vi "Dashboard Main.vi"() -> ()   [LabVIEW 2015]
uses:
  <vilib>/Utility/miscctls.llb/LVRowAndColumnTypeDef.ctl
  <vilib>/event_ctls.llb/eventvkey.ctl
  <vilib>/Rock Robotics/WPI/Dashboard/WPI_DashboardLogging Global.vi
  <vilib>/Rock Robotics/Network Tables/NT Read Boolean.vi
  <vilib>/Rock Robotics/Network Tables/NT Write Boolean.vi
  <vilib>/Utility/config.llb/Write Key (String).vi
  <vilib>/Utility/config.llb/Write Key (I32).vi
  <vilib>/Utility/config.llb/NI_LVConfig.lvlib
panel:
  out "IP Display":string
  in  "TCP":refnum<k5>
  in  "Rec Mode":enum32{"Stop", "Record", "Playback"}(radio)
  in  "Vision":u16(ring)=2 items=["Camera Off", "USB Camera SW", "USB Camera HW", "IP Camera"]
  out "Camera IP":string
  out "Image Message":string="Timeout in Camera Communications"
  in  "Dashboard Tab":T1(tab)
  out "Roll":dbl(slide) scale=0.0..359.0
  out "Pitch":dbl(slide) scale=0.0..359.0
  in  "Select Auto":string(combo)
  out "NT Connection":bool
  in  "Camera Settings":T2={"Frame Rate"=30, "Compression"=30, "Size"=1} {"Frame Rate" scale=1.0..30.0; "Size" items=["640x480", "320x240", "160x120"]}
  out "Gyro":dbl(knob) scale=0.0..360.0
  out "Mode":T3(ring)=enum."Auto Disabled"
  in  "DB Camera Config":bool
  out "fps":dbl format="%#.1g"
  out "Mbps":dbl format="%#.1g"
  out "Mbps LED":bool
  out "isLevel":bool
  out "isGoalCentered":bool
  out "isInSuckState":bool
  out "isOverDefense":bool
  out "Shooter Motors Not Spinning":bool
  out "Script Corrupt?":bool
  out "Com":dbl min=0.0 max=9.0 step=1.0
  out "Auto0":string caption="DB/String 0"
  out "Auto1":string caption="DB/String 1"
  out "Auto2":string caption="DB/String 2"
  out "Auto3":string caption="DB/String 3"
  out "Pos":dbl min=1.0 max=6.0
  out "Script Exists?":bool
  out "Roller Arm State":T4(ring)
  out "Shooter Angle State":T5(ring)
  out "Shooting State":T6(ring)
  out "RollerAngleDesired":dbl
  out "RollerAngleActual":dbl
  out "ShooterAngleDesired":dbl
  out "ShooterAngleActual":dbl
  out "WheelOneDesired":dbl
  out "WheelOneActual":dbl
  out "WheelTwoDesired":dbl
  out "WheelTwoActual":dbl
  in  "doAutoShoot":bool
  in  "ShooterGuideH":i32(slide)=170 min=0 max=320 step=1 scale=0.0..320.0
  in  "ShooterGuideV":i32(slide)=130 caption="ShooterGuide" min=0 max=240 step=1
  in  "Test Slider":dbl(slide) scale=0.0..100.0 scale format="%#_3g"
  in  "On/Off":bool caption="Solenoid"
  in  "Test Name":u16(ring) items=["Select the test to run..."]
  in  "Test Tree":string(tree)
  in  "Motor":cluster{"Value":dbl, "Enable":bool} {"Value" scale=-1.0..1.0 scale format="%#_3g"}
  out "Progress":T7 {"Test Progress" scale=0.0..100.0}
  in  "Rev/Fwd":cluster{"Forward":bool, "Reverse":bool}
  in  "Test Ring":u16(ring) items=["Monochrome", "Color"]
  out "Cmd Status":string
  in  "Execute Command":bool
  in  "Command Params":string[][](table)
  in  "Command Selection":i32(listbox)
  in  "CheckList":i32(listbox)
  out "Tree":string(tree)
  out "Camera Image":T8(plugin-control)
  out "Background":bool
  # "Pitch"
  # "Roll"
  # "D-PAD\n/\\ +Position\n\\/ - Position\n< + Command\n>  - Command"
  # "COMMANDS\n0 - Cross Defense\n1 - Cross Defense, Spit Ball, Return, Spin\n2 - Score Low - Ramp, Moat, Wall, Terrain, Low Bar\n3 - Score High - Ramp, Moat, Wall, Terrain, Low Bar\n4 - Score Low - Cheval de Frise\n5 - Score High - Cheval de Frise\n6 - Score Low - Portcullis\n7 - Score High - Portcullis\n8 - \n9 - \n\nPosition 0 Command 0 - STOP"
  # "POSITION\n0 - Test Scripts\n1 - Defense 1 Low Bar\n2 - Defense 2\n3 - Defense 3\n4 - Defense 4\n5 - Defense 5 Passage\n6 - Spy Box"
  # "Actual"
  # "Desired"
  # "WheelOne"
  # "WheelTwo"
  # "RollerAngle"
  # "ShooterAngle"
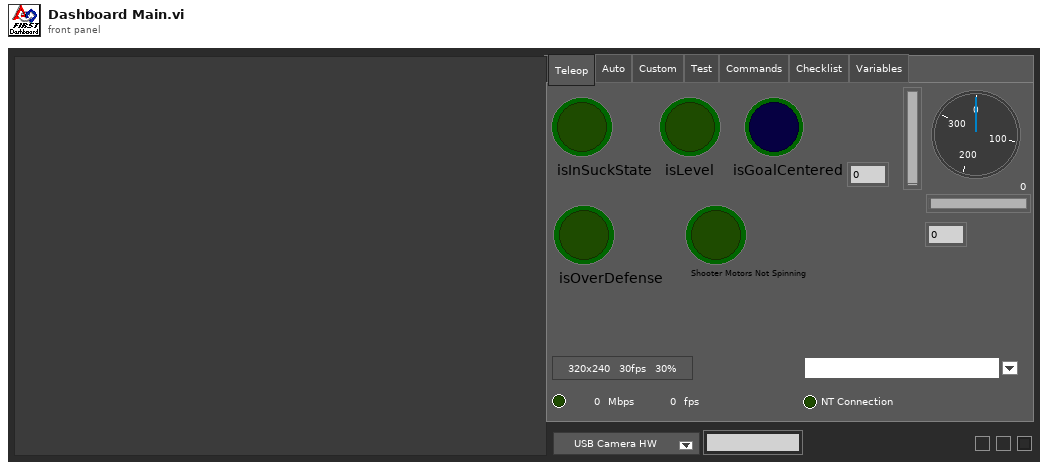
[diagram p1: front panel]
types:
  T1 = enum32{"Teleop", "Auto", "Custom", "Test", "Commands", "Checklist", "Variables"}
  T2 = cluster{"Frame Rate":i32, "Compression":i32, "Size":u16}
  T3 = enum8{"Tele-Op Disabled", "Tele-Op Enabled", "Auto Disabled", "Auto Enabled", "Test Disabled", "Test Enabled", "Disconnected", "No Code", "E-Stop"}
  T4 = enum16{"ResetBack", "EmergencyManualControl", "ResetForward", "Hold", "Reset", "ManualControl"}
  T5 = enum16{"ResetBack", "ResetForward", "Reset", "Hold", "HighGoal", "LowGoal", "BumperShot", "EmergencyManualControl"}
  T6 = enum16{"Empty", "Suck", "Hold", "LowGoal", "HighGoal", "BumperShot", "Shoot", "Dwell"}
  T7 = cluster{"Test Progress":u8, "Test Progress Text":string}
  T8 = typedef "IMAQ Image.ctl" = refnum<image>
  T9 = cluster{"IDs":cluster{"RPC field ID":u16, "Unique ID":u16}, "String":string}
  T10 = enum32{"Drive", "Basic", "Custom", "Test", "Checklist", "Variables"}
  T11 = enum32{"Teleop", "Auto", "Custom", "Test", "Checklist", "Variables"}
  T12 = typedef "Image Type" = u32
  T13 = cluster{"Camera Image":refnum<vi>, "Dashboard Tab":refnum<vi>, "Background":refnum<vi>, "Vision":refnum<vi>, "Rec Mode":refnum<vi>, "Test Slider":refnum<vi>, "On/Off ":refnum<vi>, "Test Ring":refnum<vi>, "Rev/Fwd":refnum<vi>, "Test Name":refnum<vi>, "Motor":refnum<vi>, "Progress":refnum<vi>, "CheckList":refnum<vi>, "Tree":refnum<vi>, "Test Tree":refnum<vi>, "Command Params":refnum<vi>, "Command Selection":refnum<vi>, "Execute Command":refnum<vi>, "Cmd Status":refnum<vi>}
  T14 = cluster{"Error Strings":string, "Disable Counts":cluster{u16, u16}, "Rail Faults":cluster{u16, u16, u16}, "Robot IP":string, "DB Mode":u8, "Event Info":cluster{"Name":string, "Type":u8, "Number":u16, "Replay":u8}, "Camera Addr":string}
  T15 = cluster{"Storage":cluster{"Disk Free":u64, "RAM Block":u32, "RAM free":u32}, "CPU Utilization":cluster{"CPU % ISR":sgl, "CPU % Time Crit":sgl, "CPU % Timed Str":sgl, "CPU % High":sgl, "CPU % Above":sgl, "CPU % Normal":sgl, "CPU % Low":sgl}, "CAN":cluster{"% Bus Utilization":sgl, "Bus Off Cnt":u32, "TX_FIFO Full Cnt":u32, "Receive Error Cnt":u8, "Transmit Error Cnt":u8}, "HID":cluster{"HID Outputs":u32, "Rumble Low":u16, "Rumble High":u16}[]}
  T16 = cluster{"Status bits":cluster{"Test Mode":bool, "Autonomous":bool, "Enabled":bool, "Code Start":bool, "Brownout":bool, "Reserved 2":bool, "Reserved 3":bool, "E-Stop":bool}, "Code Trace":cluster{"Disabled":bool, "TeleOp":bool, "Auto":bool, "Test":bool}, "Controller Type":enum16{"unknown", "cRIO", "roboRio"}, "Code?":enum16{"unknown", "noCode", "code"}, "Battery V":dbl}
  T17 = cluster{"Control Bits":cluster{"TestMode":bool, "Autonomous":bool, "Enabled":bool, "FMS Present":bool, bool, bool, bool, "E-Stop":bool}, "Team Station ":u8, "Countdown":sgl, "Joystick Values":cluster{"Axes":dbl[], "Buttons":bool[], "POVs":i16[]}[]}
  T18 = typedef "NI_LVConfig.lvlib/Config Data RefNum.ctl" = refnum<k1>
  T19 = cluster{"Operation":enum16{"Update", "Clear"}, "Color Box":u32}[]
  T20 = typedef "eventvkey.ctl" = enum16{"ASCII", "Enter", "Return", "Shift", "Ctrl", "Alt", "Cmd", "Opt", "Caps", "NumLock", "Clear", "Break", "Up", "Down", "Left", "Right", "Insert", "Delete", "Home", "End", "PageUp", "PageDown", "Escape", "Help", "Pause", "ScrollLock", "F1", "F2", "F3", "F4", "F5", "F6", "F7", "F8", "F9", "F10", "F11", "F12", "F13", "F14", "F15", "F16", "F17", "F18", "F19", "F20", "F21", "F22", "F23", "F24", "Play", "VolumeUp", "VolumeDown", "Mute", "Two Byte Char"}
  T21 = cluster{"Image Size":bool, "Image Type":bool, "Pixel Value":bool, "ROI Information":bool, "Zoom Factor":bool}
  T22 = enum8{"Enabled", "Disabled", "Disabled and Grayed Out"}
  T23 = cluster{"Operation":enum16{"Update", "Clear"}, "Color Box":u32}
  T24 = typedef "LVRowAndColumnTypeDef.ctl" = cluster{"Row":i32, "Column":i32}
  T25 = cluster{"Shift":bool, "Ctrl":bool, "Alt":bool, "Cmd":bool, "Opt":bool}
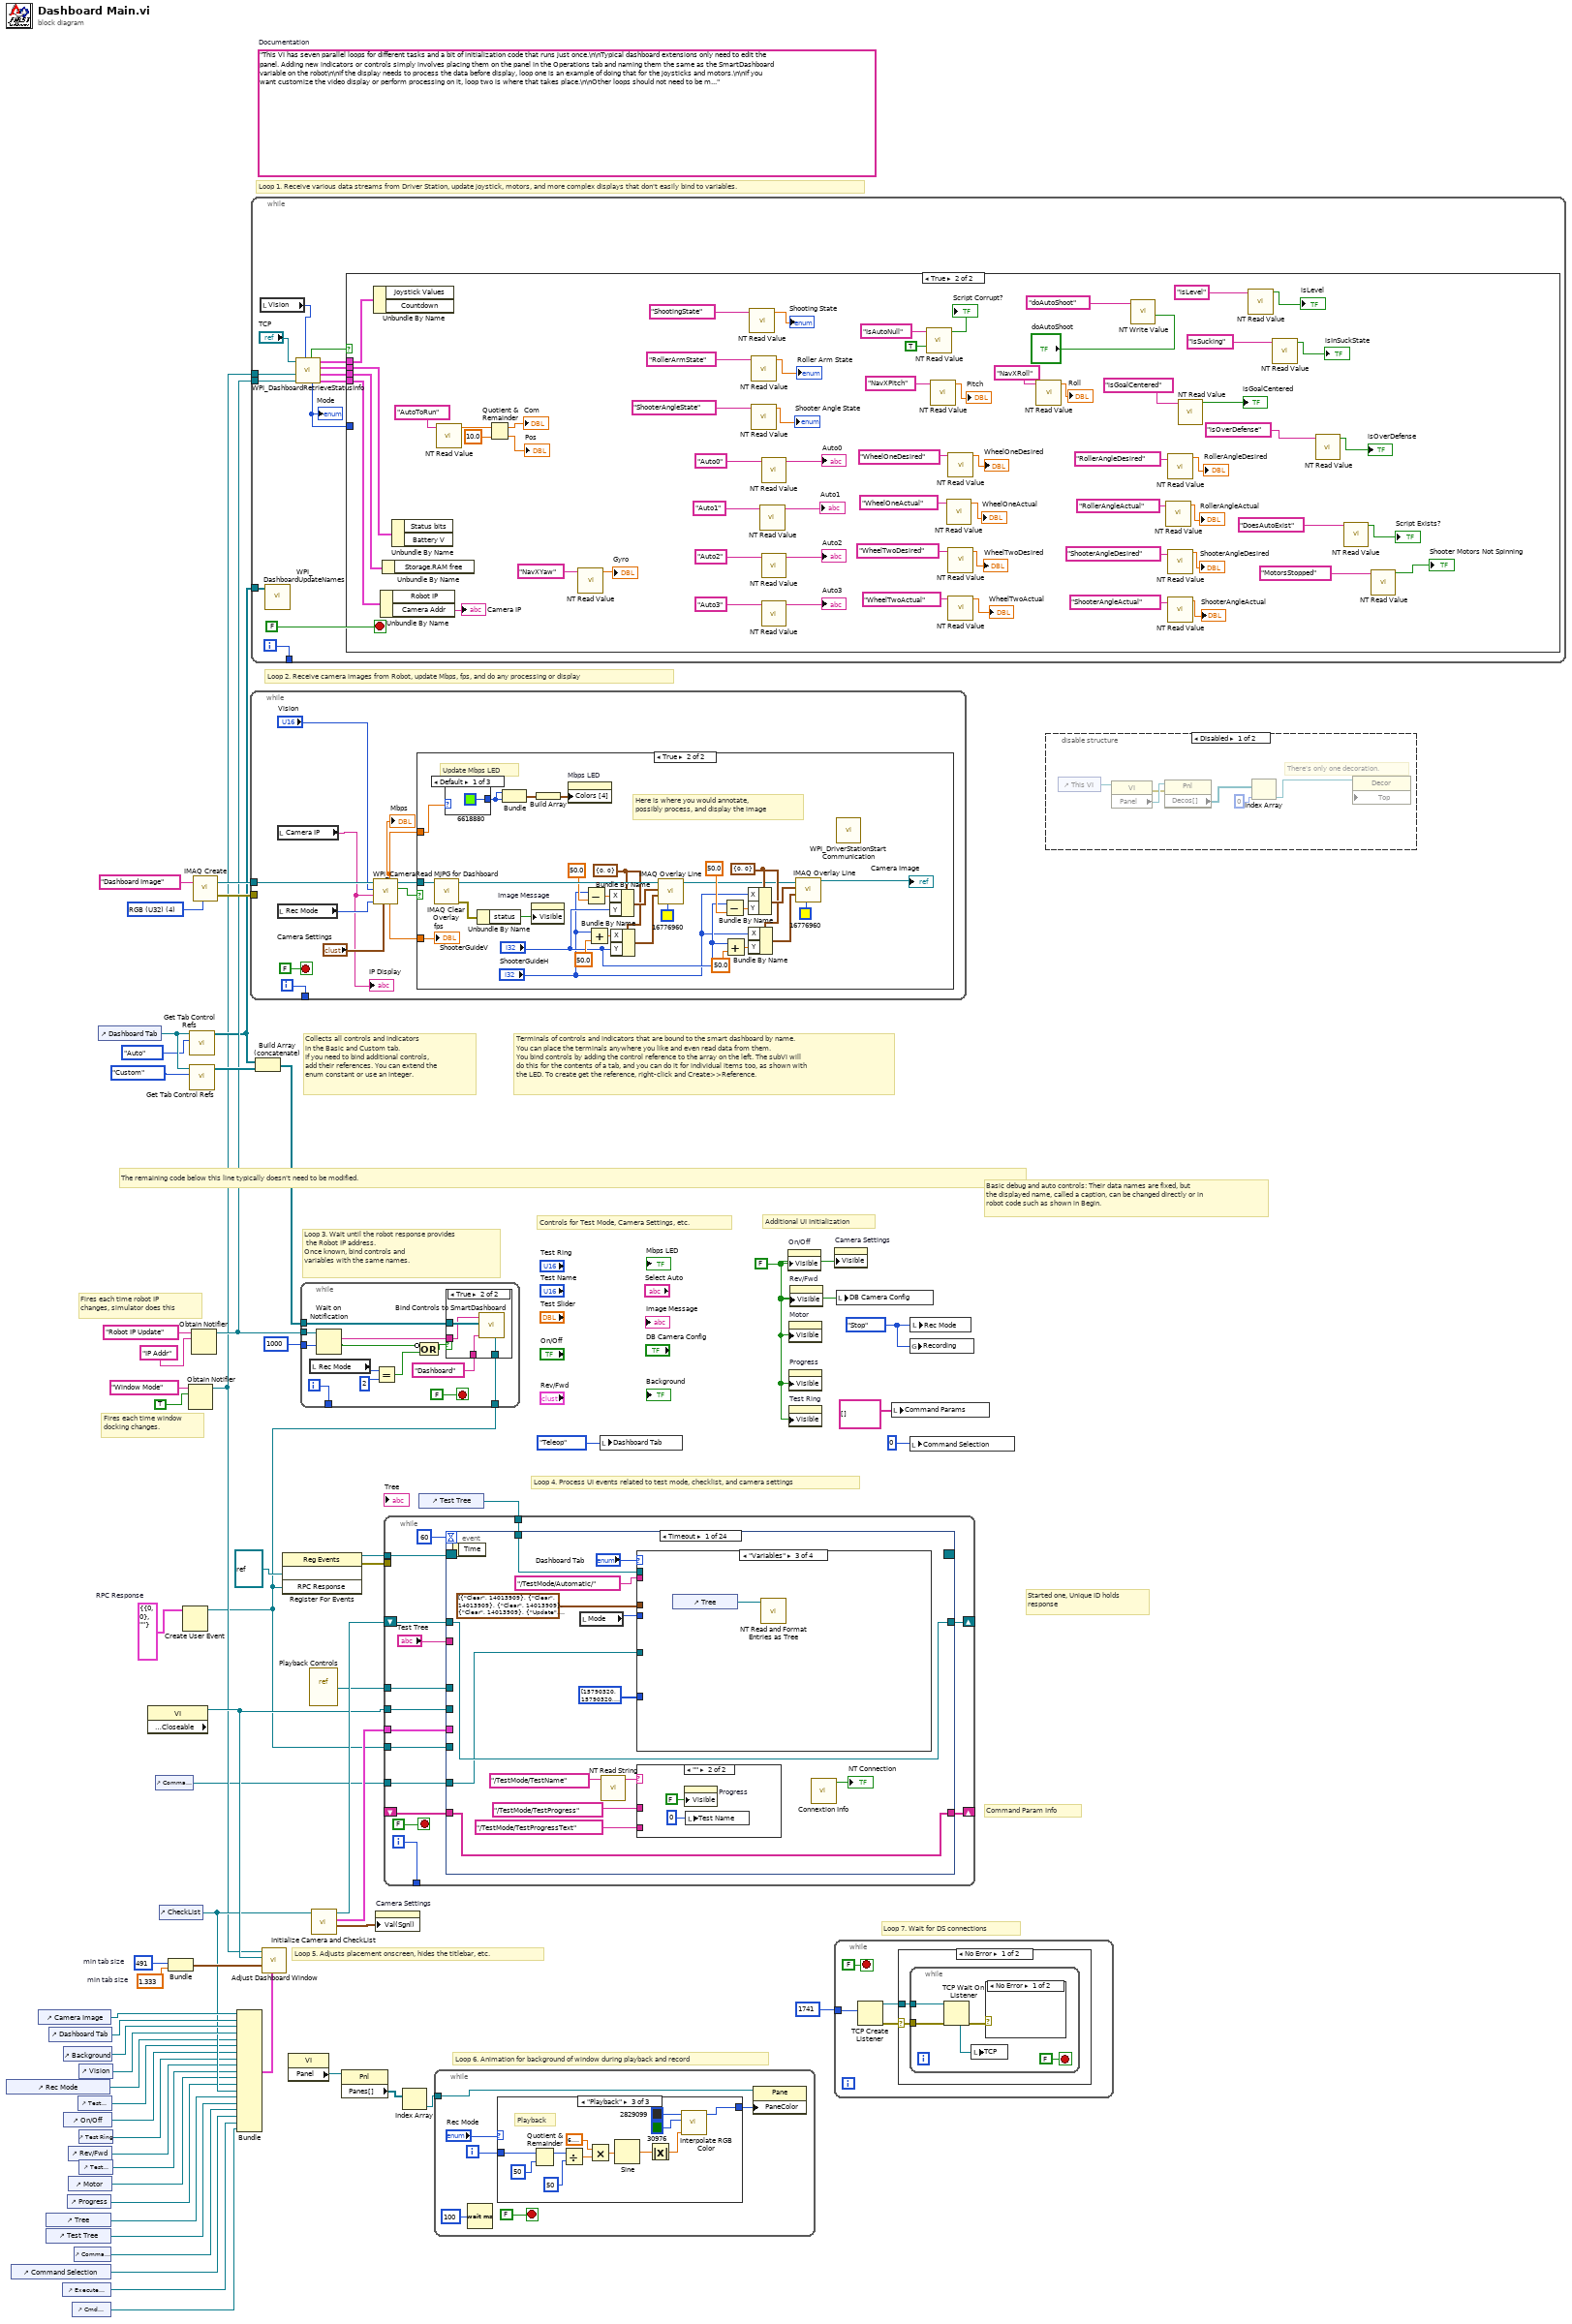
[diagram p0: block diagram]
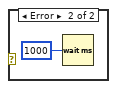
[diagram p3: hidden frame]
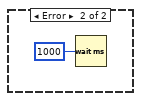
[diagram p4: hidden frame]
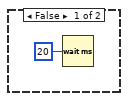
[diagram p5: hidden frame]
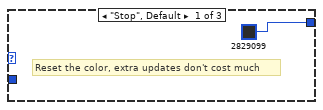
[diagram p6: hidden frame]
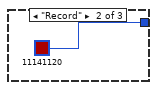
[diagram p7: hidden frame]
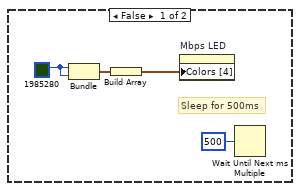
[diagram p9: hidden frame]
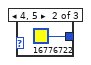
[diagram p10: hidden frame]
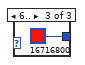
[diagram p11: hidden frame]
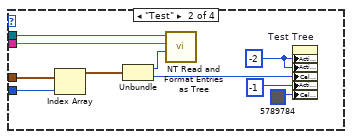
[diagram p13: hidden frame]
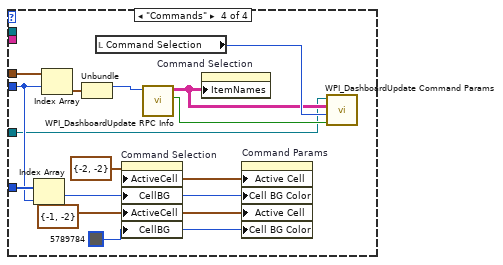
[diagram p14: hidden frame]
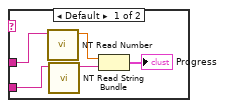
[diagram p15: hidden frame]
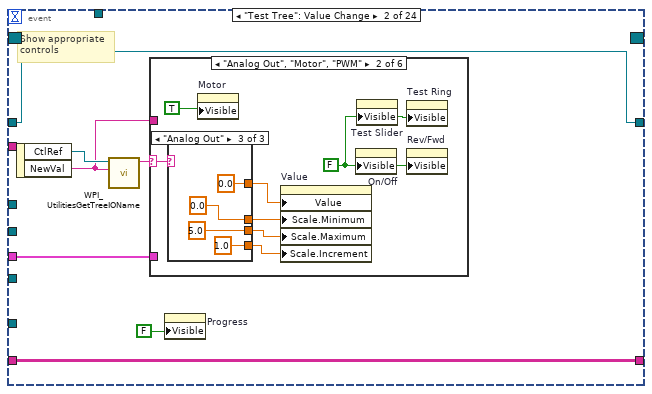
[diagram p16: hidden frame]
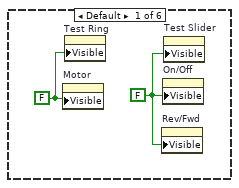
[diagram p17: hidden frame]
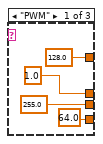
[diagram p18: hidden frame]
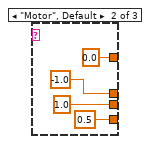
[diagram p19: hidden frame]
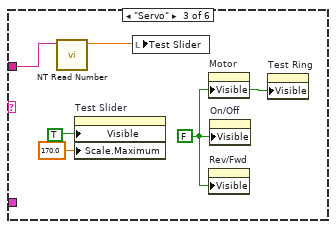
[diagram p20: hidden frame]
diagram:
  w7 = T9 {"IDs"={"RPC field ID"=0, "Unique ID"=0}, "String"=""}  # RPC Response
  w33 = 491  # min tab size
  w32 = 1.333  # min tab size
  w41 = enum32{"Stop", "Record", "Playback"}."Stop" ("Rec Mode")
  w15 = FALSE ("Visible")
  (unwired) "This VI has seven parallel loops for different tasks and a bit of initialization code that runs just once.\n\nTypical dashboard extensions only need to edit the panel. Adding new indicators or controls simply involves placing them on the panel in the Operations tab and naming them the same as the SmartDashboard variable on the robot\n\nIf the display needs to process the data before display, loop one is an example of doing that for the joysticks and motors.\n\nIf you want customize the video display or perform processing on it, loop two is where that takes place.\n\nOther loops should not need to be modified. They are pretty standard, and document the task they perform."  # Documentation
  w61 = T12 4 items=["Grayscale (U8)", "Grayscale (I16)", "Grayscale (SGL)", "Complex (CSG)", "RGB (U32)", "HSL (U32)", "RGB (U64)"] ("Image Type")
  # "Command Param Info"
  # "Started one, Unique ID holds\nresponse"
  # "Loop 7. Wait for DS connections"
  # "Basic debug and auto controls: Their data names are fixed, but\nthe displayed name, called a caption, can be changed directly or in\nrobot code such as shown in Begin."
  # "Controls for Test Mode, Camera Settings, etc."
  # "Additional UI Initialization"
  # "Loop 6. Animation for background of window during playback and record"
  # "Fires each time robot IP\nchanges, simulator does this"
  # "Fires each time window\ndocking changes."
  # "Collects all controls and indicators\nin the Basic and Custom tab.\nIf you need to bind additional controls,\nadd their references. You can extend the\nenum constant or use an integer."
  # "The remaining code below this line typically doesn't need to be modified."
  # "Loop 4. Process UI events related to test mode, checklist, and camera settings"
  # "Terminals of controls and indicators that are bound to the smart dashboard by name.\nYou can place the terminals anywhere you like and even read data from them.\nYou bind controls by adding the control reference to the array on the left. The subVI will\ndo this for the contents of a tab, and you can do it for individual items too, as shown with\nthe LED. To create get the reference, right-click and Create>>Reference."
  # "Loop 3. Wait until the robot response provides\n the Robot IP address.\nOnce known, bind controls and\nvariables with the same names."
  # "Loop 5. Adjusts placement onscreen, hides the titlebar, etc."
  # "Loop 1. Receive various data streams from Driver Station, update joystick, motors, and more complex displays that don't easily bind to variables."
  # "Loop 2. Receive camera images from Robot, update Mbps, fps, and do any processing or display"
  n1 = control-ref of="Rec Mode"() -> (w21:refnum<vi>)
  n2 = control-ref of="Command Selection"() -> (w6:refnum<vi>)
  n3 = control-ref of="Camera Image"() -> (w36:refnum<vi>)
  n4 = control-ref of="Tree"() -> (w25:refnum<vi>)
  n5 = control-ref of="Test Tree"() -> (w24:refnum<vi>)
  n6 = control-ref of="Dashboard Tab"() -> (w35:refnum<vi>)
  n7 = control-ref of="Execute Command"() -> (w8:refnum<vi>)
  n8 = control-ref of="Background"() -> (w30:refnum<vi>)
  n9 = control-ref of="On/Off"() -> (w19:refnum<vi>)
  n10 = control-ref of="Progress"() -> (w16:refnum<vi>)
  n11 = control-ref of="Rev/Fwd"() -> (w17:refnum<vi>)
  n12 = control-ref of="Motor"() -> (w22:refnum<vi>)
  n13 = control-ref of="Cmd Status"() -> (w2:refnum<vi>)
  n14 = control-ref of="Command Params"() -> (w9:refnum<vi>)
  n15 = control-ref of="Test Slider"() -> (w20:refnum<vi>)
  n16 = control-ref of="Vision"() -> (w34:refnum<vi>)
  n17 = control-ref of="Test Ring"() -> (w18:refnum<vi>)
  n18 = control-ref of="Test Name"() -> (w23:refnum<vi>)
  n19 = control-ref of="Dashboard Tab"() -> (w39:refnum<vi>)
  n20 = property class="VI" props=["Front Panel.Closeable"]() -> (reference out=w40:refnum<vi>)  [unwired: 2 in, 2 out]
  n21 = control-ref of="Command Params"() -> (w1:refnum<vi>)
  n22 = control-ref of="CheckList"() -> (w26:refnum<vi>)
  n23 = Bundle("min tab size"=w33, "min tab size"=w32) -> (w31:cluster{"min tab size":i32, "min tab size":dbl})  [unwired: 1 in]
  n24 = Create User Event(user event datatype=w7) -> (user event=w3:refnum<user-event>)  [unwired: 1 in, 1 out]
  n25 = Obtain Notifier(name (unnamed)="Window Mode", notification data type=TRUE) -> (notifier out=w12:refnum<notifier>)  [unwired: 2 in, 2 out]
  n26 = call <vilib>:"Get Tab Control Refs.vi"("Page Index"=T11."Auto" ("Dashboard Tab"), "TabControl in"=w39) -> ("ControlsOnPage"=w13:refnum<vi>[])  [unwired: 9 in]
  n27 = call <vilib>:"Get Tab Control Refs.vi"("Page Index"=T10."Custom" ("Dashboard Tab"), "TabControl in"=w39) -> ("ControlsOnPage"=w38:refnum<vi>[])  [unwired: 9 in]
  n28 = Obtain Notifier(name (unnamed)="Robot IP Update", notification data type="IP Addr" ("name (unnamed)")) -> (notifier out=w14:refnum<notifier>)  [unwired: 2 in, 2 out]
  n29 = call "IMAQ Create"("Image Name"="Dashboard Image", "Image Type"=w61) -> ("New Image"=w59:T8, "error out"=w58:errorcluster)  [unwired: 2 in, 1 out]
  n30 = Bundle("Camera Image"=w36, "Dashboard Tab"=w35, "Background"=w30, "Vision"=w34, "Rec Mode"=w21, "Test Slider"=w20, "On/Off"=w19, "Test Ring"=w18, "Rev/Fwd"=w17, "Test Name"=w23, "Motor"=w22, "Progress"=w16, "CheckList"=w26, "Tree"=w25, "Test Tree"=w24, "Command Params"=w9, "Command Selection"=w6, "Execute Command"=w8, "Cmd Status"=w2) -> (w27:T13)  [unwired: 1 in]
  n31 = while {
    tunnel: w59 -> [w70]
    tunnel: w58 -> [_]
    tunnel: [w71] -> _
    i -> [w71]
    stop <- FALSE stop-if-true
    n32 = local read "Camera IP"() -> (w62:string)
    "IP Display" <- w62
    n33 = local read "Rec Mode"() -> (w65:enum32{"Stop", "Record", "Playback"})
    n34 = call <vilib>:"WPI_CameraRead MJPG for Dashboard.vi"("Camera Settings"="Camera Settings", "Rec Mode"=w65, "Camera IP"=w62, "Camera Mode"="Vision", "Refnum in"=w70) -> ("Active"=w68:bool, "Refnum out"=w69:T8, "FPS"=w67:dbl, "Bandwidth (Mbps)"=w64:dbl)  [unwired: 3 in]
    "Mbps" <- w64
    n35 = case shown="True" w68 {
      tunnel: w69 -> [_ w100]
      tunnel: w64 -> [_ w99]
      tunnel: w67 -> [_ w98]
      frame False {
        w73 = u32 1985280 ("Color Box")
        # "Sleep for 500ms"
        n36 = Bundle("Color Box"=w73, "Color Box"=w73) -> (w75:cluster{"Color Box":u32, "Color Box":u32})  [unwired: 1 out]
        n37 = Build Array(w75) -> (w74:cluster{"Color Box":u32, "Color Box":u32}[])
        n38 = property on="Mbps LED" class="Bool (strict)"("Colors [4]"=w74) -> ()  [unwired: 2 in, 2 out]
        n39 = Wait Until Next ms Multiple(millisecond multiple=u32 500) -> ()  [unwired: 1 out]
      }
      frame True {
        w86 = cluster{"X":i32, "Y":i32} {"X"=0, "Y"=0} ("Start Point")
        w94 = cluster{"X":i32, "Y":i32} {"X"=0, "Y"=0} ("Start Point")
        # "Here is where you would annotate,\npossibly process, and display the image"
        # "Update Mbps LED"
        n40 = call "IMAQ Clear Overlay"("Image"=w100) -> ("error out"=w104:errorcluster, "Image Out"=w97:T8)  [unwired: 2 in, 7 out]
        n41 = case shown="Default" w99 {
          tunnel: [u32 6618880 ("Color Box") u32 16776722 ("Color Box") u32 16716800 ("Color Box")] -> w101
          frame Default {
          }
          frame 4, 5 {
          }
          frame 6.. {
          }
        }
        n42 = Unbundle By Name(w104) -> ("status"=w105:bool)
        n43 = Bundle("Color Box"=w101, "Color Box"=w101) -> (w103:cluster{"Color Box":u32, "Color Box":u32})  [unwired: 1 out]
        n44 = property on="Image Message" class="Str"("Visible"=w105) -> ()  [unwired: 2 in, 2 out]
        n45 = Build Array(w103) -> (w102:cluster{"Color Box":u32, "Color Box":u32}[])
        n46 = property on="Mbps LED" class="Bool (strict)"("Colors [4]"=w102) -> ()  [unwired: 2 in, 2 out]
        n47 = Subtract(x="ShooterGuideH", y=50.0) -> (x-y=w92:dbl)
        n48 = Add(x="ShooterGuideH", y=50.0) -> (x+y=w91:dbl)
        n49 = Bundle By Name(cluster=w94, "X"=w92, "Y"="ShooterGuideV") -> (w96:cluster{"X":i32, "Y":i32})
        n50 = Bundle By Name(cluster=w94, "X"=w91, "Y"="ShooterGuideV") -> (w95:cluster{"X":i32, "Y":i32})
        n51 = call "IMAQ Overlay Line"("Color"=u32 16776960, "End Point"=w95, "Start Point"=w96, "Image"=w97) -> ("Image Out"=w82:T8)  [unwired: 6 in, 1 out]
        n52 = Subtract(x="ShooterGuideV", y=50.0) -> (x-y=w81:dbl)
        n53 = Add(x="ShooterGuideV", y=50.0) -> (x+y=w79:dbl)
        n54 = Bundle By Name(cluster=w86, "X"="ShooterGuideH", "Y"=w81) -> (w88:cluster{"X":i32, "Y":i32})
        n55 = Bundle By Name(cluster=w86, "X"="ShooterGuideH", "Y"=w79) -> (w87:cluster{"X":i32, "Y":i32})
        n56 = call "IMAQ Overlay Line"("Color"=u32 16776960, "End Point"=w87, "Start Point"=w88, "Image"=w82) -> ("Image Out"=→"Camera Image":T8)  [unwired: 6 in, 1 out]
        n57 = call <vilib>:"WPI_DriverStationStart Communication.vi"() -> ()  [unwired: 12 in]
        "fps" <- w98
      }
    }
  }
  n58 = while {
    tunnel: [w120] -> _
    tunnel: w14 -> [w114]
    tunnel: w13 -> [w113]
    tunnel: w12 -> [w109]
    i -> [w120]
    stop <- FALSE stop-if-true
    n59 = local read "Vision"() -> (w111:u16)
    n60 = call <vilib>:"WPI_DashboardUpdateNames.vi"("Controls on Tab"=w113) -> ()  [unwired: 11 in]
    n61 = call <vilib>:"WPI_DashboardRetrieveStatusInfo.vi"("Vision"=w111, "Binding Refnum"=w114, "Window Mode Notifier"=w109, "TCP Cnx"="TCP") -> ("Power and Errors"=w115:T14, "Robot Metrics"=w118:T15, "Status Info"=w119:T16, "Control Info"=w116:T17, "Robot Mode"=w112:T3, "Process?"=w117:bool)  [unwired: 2 in]
    "Mode" <- w112
    n62 = case shown="True" w117 {
      tunnel: w119 -> [_ w185]
      tunnel: w118 -> [_ w184]
      tunnel: w116 -> [_ w183]
      tunnel: w115 -> [_ w182]
      tunnel: w112 -> [_ _]
      frame False {
        n63 = Wait (ms)(milliseconds to wait=u32 20) -> ()  [unwired: 1 out]
      }
      frame True {
        n64 = Unbundle By Name(w183) -> ()  [unwired: 2 out]
        n65 = Unbundle By Name(w182) -> ("Camera Addr"=→"Camera IP":string)  [unwired: 1 out]
        n66 = Unbundle By Name(w184) -> ()  [unwired: 1 out]
        n67 = Unbundle By Name(w185) -> ()  [unwired: 2 out]
        n68 = call-poly <vilib>:"NT Read Value.vi"("Name"="AutoToRun") -> ("Numeric"=w131:dbl)  [unwired: 9 in, 1 out]
        n69 = Quotient & Remainder(x=w131, y=10.0) -> (x-y*floor(x/y)=→"Com":dbl, floor(x/y)=→"Pos":dbl)
        n70 = call-poly <vilib>:"NT Read Value.vi"("Name"="NavXYaw") -> ("Numeric"=→"Gyro":dbl)  [unwired: 9 in, 1 out]
        n71 = call-poly <vilib>:"NT Read Value.vi"("Name"="ShootingState") -> ("Numeric"=→"Shooting State":dbl)  [unwired: 9 in, 1 out]
        n72 = call-poly <vilib>:"NT Read Value.vi"("Name"="RollerArmState") -> ("Numeric"=→"Roller Arm State":dbl)  [unwired: 9 in, 1 out]
        n73 = call-poly <vilib>:"NT Read Value.vi"("Name"="ShooterAngleState") -> ("Numeric"=→"Shooter Angle State":dbl)  [unwired: 9 in, 1 out]
        n74 = call-poly <vilib>:"NT Read Value.vi"("Name"="Auto1") -> ("String"=→"Auto1":string)  [unwired: 9 in, 1 out]
        n75 = call-poly <vilib>:"NT Read Value.vi"("Name"="Auto0") -> ("String"=→"Auto0":string)  [unwired: 9 in, 1 out]
        n76 = call-poly <vilib>:"NT Read Value.vi"("Name"="Auto2") -> ("String"=→"Auto2":string)  [unwired: 9 in, 1 out]
        n77 = call-poly <vilib>:"NT Read Value.vi"("Name"="Auto3") -> ("String"=→"Auto3":string)  [unwired: 9 in, 1 out]
        n78 = call-poly <vilib>:"NT Read Value.vi"("Default Value"=TRUE, "Name"="IsAutoNull") -> ("Boolean"=→"Script Corrupt?":bool)  [unwired: 8 in, 1 out]
        n79 = call-poly <vilib>:"NT Read Value.vi"("Name"="NavXPitch") -> ("Numeric"=→"Pitch":dbl)  [unwired: 9 in, 1 out]
        n80 = call-poly <vilib>:"NT Read Value.vi"("Name"="WheelOneActual") -> ("Numeric"=→"WheelOneActual":dbl)  [unwired: 9 in, 1 out]
        n81 = call-poly <vilib>:"NT Read Value.vi"("Name"="WheelOneDesired") -> ("Numeric"=→"WheelOneDesired":dbl)  [unwired: 9 in, 1 out]
        n82 = call-poly <vilib>:"NT Read Value.vi"("Name"="WheelTwoDesired") -> ("Numeric"=→"WheelTwoDesired":dbl)  [unwired: 9 in, 1 out]
        n83 = call-poly <vilib>:"NT Read Value.vi"("Name"="WheelTwoActual") -> ("Numeric"=→"WheelTwoActual":dbl)  [unwired: 9 in, 1 out]
        n84 = call-poly <vilib>:"NT Read Value.vi"("Name"="NavXRoll") -> ("Numeric"=→"Roll":dbl)  [unwired: 9 in, 1 out]
        n85 = call-poly <vilib>:"NT Write Value.vi"("Boolean"="doAutoShoot", "Name"="doAutoShoot") -> ()  [unwired: 9 in, 1 out]
        n86 = call-poly <vilib>:"NT Read Value.vi"("Name"="RollerAngleActual") -> ("Numeric"=→"RollerAngleActual":dbl)  [unwired: 9 in, 1 out]
        n87 = call-poly <vilib>:"NT Read Value.vi"("Name"="RollerAngleDesired") -> ("Numeric"=→"RollerAngleDesired":dbl)  [unwired: 9 in, 1 out]
        n88 = call-poly <vilib>:"NT Read Value.vi"("Name"="ShooterAngleDesired") -> ("Numeric"=→"ShooterAngleDesired":dbl)  [unwired: 9 in, 1 out]
        n89 = call-poly <vilib>:"NT Read Value.vi"("Name"="ShooterAngleActual") -> ("Numeric"=→"ShooterAngleActual":dbl)  [unwired: 9 in, 1 out]
        n90 = call-poly <vilib>:"NT Read Value.vi"("Name"="isGoalCentered") -> ("Boolean"=→"isGoalCentered":bool)  [unwired: 9 in, 1 out]
        n91 = call-poly <vilib>:"NT Read Value.vi"("Name"="isLevel") -> ("Boolean"=→"isLevel":bool)  [unwired: 9 in, 1 out]
        n92 = call-poly <vilib>:"NT Read Value.vi"("Name"="isSucking") -> ("Boolean"=→"isInSuckState":bool)  [unwired: 9 in, 1 out]
        n93 = call-poly <vilib>:"NT Read Value.vi"("Name"="isOverDefense") -> ("Boolean"=→"isOverDefense":bool)  [unwired: 9 in, 1 out]
        n94 = call-poly <vilib>:"NT Read Value.vi"("Name"="DoesAutoExist") -> ("Boolean"=→"Script Exists?":bool)  [unwired: 9 in, 1 out]
        n95 = call-poly <vilib>:"NT Read Value.vi"("Name"="MotorsStopped") -> ("Boolean"=→"Shooter Motors Not Spinning":bool)  [unwired: 9 in, 1 out]
      }
    }
  }
  n96 = Build Array (concatenate)(w13, w38) -> (w37:refnum<vi>[])
  n97 = call "Adjust Dashboard Window.vi"("Sizing Refnums"=w27, "Size Constraints"=w31, "VI"=w40, "WIn Mode"=w12) -> ()  [unwired: 8 in]
  n98 = register-events(refnum<vi> refnum, w3) -> (reference out=w45:refnum<event-registration>, error out=w44:errorcluster)  [unwired: 2 in]
  n99 = property class="VI"() -> ("Panel"=w48:refnum<vi>)  [unwired: 2 in, 2 out]
  n100 = while {
    tunnel: w37 -> [w198]
    tunnel: w14 -> [w196]
    tunnel: [w194] -> _
    tunnel: u32 1000 ("milliseconds to wait") -> [w193]
    tunnel: w3 -> [w186]
    i -> [w194]
    stop <- FALSE stop-if-true
    n101 = local read "Rec Mode"() -> (w189:enum32{"Stop", "Record", "Playback"})
    n102 = Wait on Notification(notifier=w196, timeout in ms (-1)=w193) -> (notification=w195:string, timed out?=w191:bool)  [unwired: 2 in, 2 out]
    n103 = Equal?(x=w189, y=u16 2 ("Rec Mode")) -> (x = y?=w190:bool)
    n104 = Compound Arithmetic op=OR(invert w191, w190) -> (w192:bool)
    n105 = case shown="True" w192 {
      tunnel: w198 -> [_ w202]
      tunnel: w195 -> [_ w201]
      tunnel: "Dashboard" -> [_ w200]
      tunnel: w186 -> [_ w199]
      frame False {
      }
      frame True {
        n106 = call <vilib>:"Bind Controls to SmartDashboard.vi"("RPC ref"=w199, "Client Name"=w200, "Bound Control Refs"=w202, "Server IP Address"=w201) -> ()  [unwired: 8 in]
      }
    }
  }
  n107 = vi-ref "Playback Controls.vi"() -> (w46:refnum<vi>)
  n108 = call "Initialize Camera and CheckList.vi"("ListBox in"=w26) -> ("Cluster"=w52:cluster{"value":i32, "value":i32, "index":i32}, "Array"=w53:cluster{string[]}[], "File Refnum"=w51:T18)  [unwired: 8 in]
  n109 = property class="Pnl"(reference=w48) -> ("Panes[]"=w49:refnum<vi>[])  [unwired: 1 in, 2 out]
  n110 = property on="Camera Settings" class="Clust (strict)"("Val(Sgnl)"=w52) -> ()  [unwired: 2 in, 2 out]
  n111 = Index Array(array=w49) -> (element=w47:refnum<vi>)  [unwired: 1 in]
  n112 = control-ref of="Test Tree"() -> (w50:refnum<vi>)
  n113 = while {
    tunnel: w53 -> [w214]
    shift-right: [w213] -> _
    shift-left: w51 -> [w212]
    tunnel: [w211] -> _
    tunnel: w50 -> [w210]
    tunnel: w46 -> [w209]
    tunnel: w45 -> [w208]
    tunnel: w44 -> [_]
    tunnel: w40 -> [w207]
    tunnel: w3 -> [w206]
    tunnel: w1 -> [w205]
    shift-right: [w204] -> _
    shift-left: _ -> [w203]
    i -> [w211]
    stop <- FALSE stop-if-true
    n114 = event shown="[0] Timeout" {
      selector: w208 -> [_ _ _ _ _ _ _ _ _ _ _ _ _ _ _ _ _ _ _ _ _ _ _ _]
      dyn-events: [_ _ _ _ _ _ _ _ _ _ _ _ _ _ _ _ _ _ w523 _ _ _ _ _] -> _
      timeout: u32 60 ("milliseconds to wait") -> [_ _ _ _ _ _ _ _ _ _ _ _ _ _ _ _ _ _ _ _ _ _ _ _]
      tunnel: w210 -> [w227 _ _ _ _ _ _ _ _ _ _ _ _ _ _ _ _ _ _ _ _ _ _ _]
      tunnel: "Test Tree" -> [_ _ _ _ _ _ _ _ _ _ _ _ _ w486 w495 w498 w503 w512 _ _ _ _ _ _]
      tunnel: w214 -> [_ w265 _ _ _ _ _ _ _ _ _ w448 w479 _ _ _ _ _ _ _ _ _ _ _]
      tunnel: [w224 w264 w368 w374 w384 w388 w394 w406 w414 w420 w433 w447 w472 w485 w493 w497 w502 w511 w525 w541 w543 w551 w562 w567] -> w213
      tunnel: w212 -> [w224 w264 w368 w374 w384 w388 w394 w406 w414 w420 w433 w446 w472 w485 w493 w497 w502 w511 w525 w541 w543 w551 w562 w567]
      tunnel: w209 -> [_ _ _ _ _ _ _ _ _ _ _ _ _ _ _ _ _ _ w526 _ w546 _ _ _]
      tunnel: w207 -> [_ _ _ _ _ _ _ _ _ _ _ _ _ _ _ _ _ _ w521 _ _ _ _ _]
      tunnel: w206 -> [_ _ _ _ _ _ _ _ _ _ _ _ _ _ _ _ _ _ w517 _ _ _ _ _]
      tunnel: w205 -> [w219 _ _ _ _ _ w392 _ _ _ _ _ _ _ _ _ _ _ _ _ _ _ _ _]
      tunnel: [w218 w263 w367 w373 w383 w389 w390 w400 w411 w419 w432 w445 w471 w484 w492 w496 w501 w510 w516 w539 w542 w547 w555 w568] -> w204
      tunnel: w203 -> [w218 w263 w367 w373 w383 w389 w390 _ _ w419 w432 w445 w471 w484 w492 w496 w501 w510 w516 w539 w542 w547 w555 w568]
      event Timeout {
        n115 = event-data() -> ()  [unwired: 1 in, 1 out]
        n116 = local read "Mode"() -> (w221:T3)
        n117 = call <vilib>:"NT Read String.vi"("Name"="/TestMode/TestName") -> ("String"=w230:string)  [unwired: 9 in, 1 out]
        n118 = case shown="\"Variables\"" "Dashboard Tab" {
          tunnel: w227 -> [_ w241 _ _]
          tunnel: "/TestMode/Automatic/" ("Name Pattern") -> [_ w240 _ _]
          tunnel: T19 [{"Operation"=enum."Clear", "Color Box"=14013909}, {"Operation"=enum."Clear", "Color Box"=14013909}, {"Operation"=enum."Clear", "Color Box"=14013909}, {"Operation"=enum."Clear", "Color Box"=14013909}, {"Operation"=enum."Update", "Color Box"=14013909}, {"Operation"=enum."Update", "Color Box"=16777215}, {"Operation"=enum."Clear", "Color Box"=14013909}, {"Operation"=enum."Clear", "Color Box"=14013909}, {"Operation"=enum."Clear", "Color Box"=14013909}] -> [_ w233 _ w250]
          tunnel: w221 -> [_ w232 _ w249]
          tunnel: u32[] [15790320, 15790320, 15790320, 15790320, 16777215, 16777215, 15790320, 15790320, 15790320] -> [_ _ _ w255]
          tunnel: w219 -> [_ _ _ w243]
          frame "Custom", Default {
          }
          frame "Test" {
            w239 = -2 ("Active Item:Row Number")
            n119 = Index Array(array=w233, index=w232) -> (element=w234:T23)
            n120 = Unbundle(w234) -> ("Operation"=w235:enum16{"Update", "Clear"}, "Color Box"=w236:u32)
            n121 = call <vilib>:"NT Read and Format Entries as Tree.vi"("Operation"=w235, "Name Pattern"=w240, "Tree Refnum"=w241) -> ()  [unwired: 7 in, 2 out]
            n122 = property on="Test Tree" class="Tree (strict)"("Active Item Row Number"=w239, "ActiveColNum"=w239, "CellBG"=w236, "Active Item Row Number"=-1 ("Active Item:Row Number"), "CellBG"=u32 5789784 ("Color Box")) -> ()  [unwired: 2 in, 2 out]
          }
          frame "Variables" {
            n123 = control-ref of="Tree"() -> (w242:refnum<vi>)
            n124 = call <vilib>:"NT Read and Format Entries as Tree.vi"("Tree Refnum"=w242) -> ()  [unwired: 9 in, 2 out]
          }
          frame "Commands" {
            w251 = u32 5789784 ("Color Box")
            w252 = T24 {"Row"=-1, "Column"=-2} ("Active Cell:Active Cell")
            w254 = T24 {"Row"=-2, "Column"=-2} ("Active Cell:Active Cell")
            n125 = Index Array(array=w255, index=w249) -> (element=w253:u32)
            n126 = Index Array(array=w250, index=w249) -> (element=w248:T23)
            n127 = Unbundle(w248) -> ("Operation"=w247:enum16{"Update", "Clear"})  [unwired: 1 out]
            n128 = local read "Command Selection"() -> (w246:i32)
            n129 = property on="Command Selection" class="MCListbox (strict)"("ActiveCell"=w254, "CellBG"=w253, "ActiveCell"=w252, "CellBG"=w251) -> ()  [unwired: 2 in, 2 out]
            n130 = call <vilib>:"WPI_DashboardUpdate RPC Info.vi"("Operation"=w247) -> ("update"=w245:bool, "commands"=w244:string[][])  [unwired: 9 in]
            n131 = property on="Command Selection" class="MCListbox (strict)"("ItemNames"=w244) -> ()  [unwired: 2 in, 2 out]
            n132 = property on="Command Params" class="Tbl (strict)"("Active Cell"=w254, "Cell BG Color"=w253, "Active Cell"=w252, "Cell BG Color"=w251) -> ()  [unwired: 2 in, 2 out]
            n133 = call <vilib>:"WPI_DashboardUpdate Command Params.vi"("Update"=w245, "NewVal"=w246, "Commands"=w244, "Param Tbl"=w243) -> ()  [unwired: 7 in, 1 out]
          }
        }
        n134 = case shown="\"\"" w230 {
          tunnel: "/TestMode/TestProgress" ("Name") -> [w257 _]
          tunnel: "/TestMode/TestProgressText" ("Name") -> [w256 _]
          frame Default {
            n135 = call <vilib>:"NT Read Number.vi"("Name"=w257) -> ("Numeric"=w258:dbl)  [unwired: 9 in, 1 out]
            n136 = call <vilib>:"NT Read String.vi"("Name"=w256) -> ("String"=w259:string)  [unwired: 9 in, 1 out]
            n137 = Bundle("Numeric"=w258, "String"=w259) -> (→"Progress":cluster{"Numeric":dbl, "String":string})  [unwired: 1 in]
          }
          frame "" {
            n138 = property on="Progress" class="Clust (strict)"("Visible"=FALSE) -> ()  [unwired: 2 in, 2 out]
            n139 = local write "Test Name"(u16 0) -> ()
          }
        }
        n140 = call <vilib>:"Connextion Info.vi"() -> ("Connected"=→"NT Connection":bool)  [unwired: 10 in, 1 out]
      }
      event "Test Tree": Value Change {
        # "Show appropriate\ncontrols"
        n141 = event-data() -> ("CtlRef"=w268:refnum<vi>, "NewVal"=w266:string)  [unwired: 1 in]
        n142 = call <vilib>:"WPI_UtilitiesGetTreeIOName.vi"("NewVal"=w266, "TreeControl in"=w268) -> ("I/O Name"=w269:string)  [unwired: 9 in]
        n143 = case shown="\"Analog Out\", \"Motor\", \"PWM\"" w269 {
          selector: w269 -> [_ w276 _ w298 w307 _]
          tunnel: w266 -> [_ _ w295 w297 _ w314]
          tunnel: w265 -> [_ _ _ _ _ w313]
          frame Default {
            w271 = FALSE ("Visible")
            w270 = FALSE ("Visible")
            n144 = property on="Motor" class="Clust (strict)"("Visible"=w270) -> ()  [unwired: 2 in, 2 out]
            n145 = property on="Test Ring" class="Ring (strict)"("Visible"=w270) -> ()  [unwired: 2 in, 2 out]
            n146 = property on="Rev/Fwd" class="Clust (strict)"("Visible"=w271) -> ()  [unwired: 2 in, 2 out]
            n147 = property on="On/Off" class="Bool (strict)"("Visible"=w271) -> ()  [unwired: 2 in, 2 out]
            n148 = property on="Test Slider" class="Slide (strict)"("Visible"=w271) -> ()  [unwired: 2 in, 2 out]
          }
          frame "Analog Out", "Motor", "PWM" {
            w277 = FALSE ("Visible")
            n149 = case shown="\"Analog Out\"" w276 {
              tunnel: [1.0 ("Value") -1.0 ("Value") 0.0 ("Value")] -> w275
              tunnel: [255.0 ("Value") 1.0 ("Value") 5.0 ("Value")] -> w274
              tunnel: [128.0 ("Value") 0.0 ("Value") 0.0 ("Value")] -> w273
              tunnel: [64.0 ("Value") 0.5 ("Value") 1.0 ("Value")] -> w272
              frame "PWM" {
              }
              frame "Motor", Default {
              }
              frame "Analog Out" {
              }
            }
            n150 = property on="Motor" class="Clust (strict)"("Visible"=TRUE) -> ()  [unwired: 2 in, 2 out]
            n151 = property on="Value" class="Slide (strict)"("Value"=w273, "Scale.Minimum"=w275, "Scale.Maximum"=w274, "Scale.Increment"=w272) -> ()  [unwired: 2 in, 2 out]
            n152 = property on="On/Off" class="Bool (strict)"("Visible"=w277) -> ()  [unwired: 2 in, 2 out]
            n153 = property on="Test Slider" class="Slide (strict)"("Visible"=w277) -> ()  [unwired: 2 in, 2 out]
            n154 = property on="Test Ring" class="Ring (strict)"("Visible"=w277) -> ()  [unwired: 2 in, 2 out]
            n155 = property on="Rev/Fwd" class="Clust (strict)"("Visible"=w277) -> ()  [unwired: 2 in, 2 out]
          }
          frame "Servo" {
            w293 = FALSE ("Visible")
            n156 = call <vilib>:"NT Read Number.vi"("Name"=w295) -> ("Numeric"=w294:dbl)  [unwired: 9 in, 1 out]
            n157 = property on="Test Slider" class="Slide (strict)"("Visible"=TRUE, "Scale.Maximum"=170.0 ("Scale.Range:Maximum")) -> ()  [unwired: 2 in, 2 out]
            n158 = local write "Test Slider"(w294) -> ()
            n159 = property on="Motor" class="Clust (strict)"("Visible"=w293) -> ()  [unwired: 2 in, 2 out]
            n160 = property on="Rev/Fwd" class="Clust (strict)"("Visible"=w293) -> ()  [unwired: 2 in, 2 out]
            n161 = property on="On/Off" class="Bool (strict)"("Visible"=w293) -> ()  [unwired: 2 in, 2 out]
            n162 = property on="Test Ring" class="Ring (strict)"("Visible"=w293) -> ()  [unwired: 2 in, 2 out]
          }
          frame "Relay", "Solenoid" {
            w296 = FALSE ("Visible")
            n163 = property on="Motor" class="Clust (strict)"("Visible"=w296) -> ()  [unwired: 2 in, 2 out]
            n164 = property on="Test Slider" class="Slide (strict)"("Visible"=w296) -> ()  [unwired: 2 in, 2 out]
            n165 = Search and Replace String(input string=w297, search string="/Value  **", replace string="/Direction") -> (result string=w303:string)  [unwired: 5 in, 3 out]
            n166 = property on="Test Ring" class="Ring (strict)"("Visible"=w296) -> ()  [unwired: 2 in, 2 out]
            n167 = call <vilib>:"NT Read String.vi"("Name"=w303) -> ("String"=w301:string)  [unwired: 9 in, 1 out]
            n168 = Equal?(x="Both directions", y=w301) -> (x = y?=w299:bool)
            n169 = Not(x=w299) -> (.not. x?=w300:bool)
            n170 = property on="Rev/Fwd" class="Clust (strict)"("Visible"=w299) -> ()  [unwired: 2 in, 2 out]
            n171 = property on="On/Off" class="Bool (strict)"("Visible"=w300, "Caption.Text"=w298) -> ()  [unwired: 2 in, 2 out]
          }
          frame "Compressor", "Digital Out" {
            w306 = FALSE ("Visible")
            # "Get direction and finish"
            n172 = property on="Motor" class="Clust (strict)"("Visible"=w306) -> ()  [unwired: 2 in, 2 out]
            n173 = property on="Test Slider" class="Slide (strict)"("Visible"=w306) -> ()  [unwired: 2 in, 2 out]
            n174 = property on="Test Ring" class="Ring (strict)"("Visible"=w306) -> ()  [unwired: 2 in, 2 out]
            n175 = property on="On/Off" class="Bool (strict)"("Visible"=TRUE, "Caption.Text"=w307) -> ()  [unwired: 2 in, 2 out]
            n176 = property on="Rev/Fwd" class="Clust (strict)"("Visible"=FALSE) -> ()  [unwired: 2 in, 2 out]
          }
          frame "Camera" {
            n177 = call <vilib>:"Get Last Path Segment.vi"("String in"=w314) -> ("String out"=w315:string)  [unwired: 10 in]
            n178 = property on="On/Off" class="Bool (strict)"("Visible"=FALSE) -> ()  [unwired: 2 in, 2 out]
            n179 = property on="Motor" class="Clust (strict)"("Visible"=FALSE) -> ()  [unwired: 2 in, 2 out]
            n180 = property on="Rev/Fwd" class="Clust (strict)"("Visible"=FALSE) -> ()  [unwired: 2 in, 2 out]
            n181 = case shown="\"White Balance  **\"" w315 {
              tunnel: w314 -> [w321 w330 w339 w348 w357 _ w363]
              tunnel: w313 -> [w319 w327 w336 w345 w354 _ _]
              frame "Size  **" {
                n182 = Index Array(array=w319) -> (element=w318:cluster{string[]})  [unwired: 1 in]
                n183 = call <vilib>:"NT Read String.vi"("Name"=w321) -> ("String"=w320:string)  [unwired: 9 in, 1 out]
                n184 = Unbundle(w318) -> (w316:string[])
                n185 = Match First String(2:w316, 3:w320) -> (0:w317:i32)  [unwired: 1 out]
                n186 = property on="Test Ring" class="Ring (strict)"("Value"=w317, "Strings []"=w316) -> ()  [unwired: 2 in, 2 out]
                n187 = property on="Test Ring" class="Ring (strict)"("Visible"=TRUE) -> ()  [unwired: 2 in, 2 out]
                n188 = property on="Test Slider" class="Slide (strict)"("Visible"=FALSE) -> ()  [unwired: 2 in, 2 out]
              }
              frame "White Balance  **" {
                n189 = Index Array(array=w327, index=1) -> (element=w328:cluster{string[]})
                n190 = call <vilib>:"NT Read String.vi"("Name"=w330) -> ("String"=w329:string)  [unwired: 9 in, 1 out]
                n191 = Unbundle(w328) -> (w325:string[])
                n192 = Match First String(2:w325, 3:w329) -> (0:w324:i32)  [unwired: 1 out]
                n193 = property on="Test Ring" class="Ring (strict)"("Value"=w324, "Strings []"=w325) -> ()  [unwired: 2 in, 2 out]
                n194 = property on="Test Ring" class="Ring (strict)"("Visible"=TRUE) -> ()  [unwired: 2 in, 2 out]
                n195 = property on="Test Slider" class="Slide (strict)"("Visible"=FALSE) -> ()  [unwired: 2 in, 2 out]
              }
              frame "Exposure  **" {
                n196 = Index Array(array=w336, index=2) -> (element=w337:cluster{string[]})
                n197 = call <vilib>:"NT Read String.vi"("Name"=w339) -> ("String"=w338:string)  [unwired: 9 in, 1 out]
                n198 = Unbundle(w337) -> (w333:string[])
                n199 = Match First String(2:w333, 3:w338) -> (0:w334:i32)  [unwired: 1 out]
                n200 = property on="Test Ring" class="Ring (strict)"("Value"=w334, "Strings []"=w333) -> ()  [unwired: 2 in, 2 out]
                n201 = property on="Test Ring" class="Ring (strict)"("Visible"=TRUE) -> ()  [unwired: 2 in, 2 out]
                n202 = property on="Test Slider" class="Slide (strict)"("Visible"=FALSE) -> ()  [unwired: 2 in, 2 out]
              }
              frame "Exposure Priority  **" {
                n203 = Index Array(array=w345, index=3) -> (element=w346:cluster{string[]})
                n204 = call <vilib>:"NT Read String.vi"("Name"=w348) -> ("String"=w347:string)  [unwired: 9 in, 1 out]
                n205 = Unbundle(w346) -> (w342:string[])
                n206 = Match First String(2:w342, 3:w347) -> (0:w343:i32)  [unwired: 1 out]
                n207 = property on="Test Ring" class="Ring (strict)"("Value"=w343, "Strings []"=w342) -> ()  [unwired: 2 in, 2 out]
                n208 = property on="Test Ring" class="Ring (strict)"("Visible"=TRUE) -> ()  [unwired: 2 in, 2 out]
                n209 = property on="Test Slider" class="Slide (strict)"("Visible"=FALSE) -> ()  [unwired: 2 in, 2 out]
              }
              frame "Color Enable  **" {
                n210 = Index Array(array=w354, index=4) -> (element=w355:cluster{string[]})
                n211 = call <vilib>:"NT Read String.vi"("Name"=w357) -> ("String"=w356:string)  [unwired: 9 in, 1 out]
                n212 = Unbundle(w355) -> (w351:string[])
                n213 = Match First String(2:w351, 3:w356) -> (0:w352:i32)  [unwired: 1 out]
                n214 = property on="Test Ring" class="Ring (strict)"("Value"=w352, "Strings []"=w351) -> ()  [unwired: 2 in, 2 out]
                n215 = property on="Test Ring" class="Ring (strict)"("Visible"=TRUE) -> ()  [unwired: 2 in, 2 out]
                n216 = property on="Test Slider" class="Slide (strict)"("Visible"=FALSE) -> ()  [unwired: 2 in, 2 out]
              }
              frame Default {
                n217 = property on="Test Ring" class="Ring (strict)"("Visible"=FALSE) -> ()  [unwired: 2 in, 2 out]
                n218 = property on="Test Slider" class="Slide (strict)"("Visible"=FALSE) -> ()  [unwired: 2 in, 2 out]
              }
              frame "Brightness  **", "Color Level  **", "Compression  **", "FPS  **", "Sharpness  **" {
                n219 = call <vilib>:"NT Read Number.vi"("Name"=w363) -> ("Numeric"=w362:dbl)  [unwired: 9 in, 1 out]
                n220 = local write "Test Slider"(w362) -> ()
                n221 = property on="Test Slider" class="Slide (strict)"("Visible"=TRUE, "Scale.Maximum"=100.0 ("Scale.Range:Maximum")) -> ()  [unwired: 2 in, 2 out]
                n222 = property on="Test Ring" class="Ring (strict)"("Visible"=FALSE) -> ()  [unwired: 2 in, 2 out]
              }
            }
          }
        }
        n223 = property on="Progress" class="Clust (strict)"("Visible"=FALSE) -> ()  [unwired: 2 in, 2 out]
      }
      event "Test Name": Mouse Enter {
        # "Populate the ring with the list of tests"
        n224 = event-data() -> ()  [unwired: 1 in, 1 out]
        n225 = call <vilib>:"NT Read String Array.vi"("Name"="/TestMode/TestList") -> ("String Array"=w372:string[])  [unwired: 9 in, 1 out]
        n226 = Build Array (concatenate)("Select the test to run...", w372) -> (w371:string[])
        n227 = property on="Test Name" class="Ring (strict)"("Strings []"=w371) -> ()  [unwired: 2 in, 2 out]
      }
      event "Test Name": Value Change {
        w375 = FALSE ("Visible")
        # "Tell the robot the test name to run"
        n228 = event-data() -> ("NewVal"=w379:u16)  [unwired: 1 in]
        n229 = property on="Test Name" class="Ring (strict)"() -> ("Strings []"=w380:string[])  [unwired: 2 in, 2 out]
        n230 = local write "Progress"(T7 {"Test Progress"=0, "Test Progress Text"=""} ("Progress")) -> ()
        n231 = Index Array(array=w380, index=w379) -> (element=w378:string)
        n232 = call <vilib>:"NT Write String.vi"("String"=w378, "Name"="/TestMode/TestName") -> ()  [unwired: 9 in, 1 out]
        n233 = property on="Progress" class="Clust (strict)"("Visible"=TRUE) -> ()  [unwired: 2 in, 2 out]
        n234 = property on="Motor" class="Clust (strict)"("Visible"=w375) -> ()  [unwired: 2 in, 2 out]
        n235 = property on="Test Slider" class="Slide (strict)"("Visible"=w375) -> ()  [unwired: 2 in, 2 out]
        n236 = property on="On/Off" class="Bool (strict)"("Visible"=w375) -> ()  [unwired: 2 in, 2 out]
        n237 = property on="Rev/Fwd" class="Clust (strict)"("Visible"=w375) -> ()  [unwired: 2 in, 2 out]
        n238 = property on="Test Ring" class="Ring (strict)"("Visible"=w375) -> ()  [unwired: 2 in, 2 out]
      }
      event "Select Auto": Mouse Enter {
        # "Populate the combo box with the list of autonomous options"
        n239 = event-data() -> ()  [unwired: 1 in, 1 out]
        n240 = call <vilib>:"NT Read String Array.vi"("Name"="Auto List") -> ("String Array"=w382:string[])  [unwired: 9 in, 1 out]
        n241 = property on="Select Auto" class="CmbBox"("Strings[]"=w382) -> ()  [unwired: 2 in, 2 out]
      }
      event "Select Auto": Value Change {
        # "User modified the Auto Selection. Write to NT variable so robot knows."
        n242 = event-data() -> ("NewVal"=w386:string)  [unwired: 1 in]
        n243 = call <vilib>:"NT Write String.vi"("String"=w386, "Name"="Auto Selector") -> ()  [unwired: 9 in, 1 out]
      }
      event "Command Selection": Value Change {
        # "Get the params and show in table"
        n244 = event-data() -> ("NewVal"=w393:i32)  [unwired: 1 in]
        n245 = property on="Command Selection" class="MCListbox (strict)"() -> ("ItemNames"=w391:string[][])  [unwired: 2 in, 2 out]
        n246 = call <vilib>:"WPI_DashboardUpdate Command Params.vi"("NewVal"=w393, "Commands"=w391, "Param Tbl"=w392) -> ()  [unwired: 8 in, 1 out]
      }
      event "Execute Command": Value Change {
        # "Started one, Unique ID holds\nresponse"
        n247 = event-data() -> ()  [unwired: 1 in, 1 out]
        n248 = property on="Command Selection" class="MCListbox (strict)"() -> ("ItemNames"=w405:string[][])  [unwired: 2 in, 2 out]
        n249 = Index Array(array=w405, index (row)="Command Selection", index (col)=0) -> (element=w403:string)
        n250 = call <vilib>:"Invoke Commands.vi"("Command Params"="Command Params", "Function Name"=w403) -> ("Params"=w399:u8, "Started"=w398:bool)  [unwired: 7 in, 1 out]
        n251 = Array Subset(array="Command Params", length (row)=w399) -> (w400:string[][])  [unwired: 3 in]
        n252 = Select(t="Executing" ("Cmd Status"), s=w398, f="" ("Cmd Status")) -> (s? t:f=→"Cmd Status":string)
      }
      event "Command Selection": Double Click {
        n253 = event-data() -> ("Row"=w415:i32)  [unwired: 1 in]
        n254 = property on="Command Selection" class="MCListbox (strict)"() -> ("ItemNames"=w418:string[][])  [unwired: 2 in, 2 out]
        n255 = local read "Command Params"() -> (w413:string[][])
        n256 = Index Array(array=w418, index (row)=w415, index (col)=0) -> (element=w416:string)
        n257 = call <vilib>:"Invoke Commands.vi"("Command Params"=w413, "Function Name"=w416) -> ("Params"=w412:u8, "Started"=w407:bool)  [unwired: 7 in, 1 out]
        n258 = Array Subset(array=w413, length (row)=w412) -> (w411:string[][])  [unwired: 3 in]
        n259 = Select(t="Executing" ("Cmd Status"), s=w407, f="" ("Cmd Status")) -> (s? t:f=w408:string)
        n260 = local write "Cmd Status"(w408) -> ()
      }
      event "CheckList": Double Click {
        # "Shift clears all"
        # "Update symbols on the listbox"
        n261 = event-data() -> ("PlatMods.Shift"=w421:bool, "Row"=w423:i32)  [unwired: 1 in]
        n262 = case shown="True" w421 {
          tunnel: w423 -> [w427 _]
          tunnel: 1 -> [w426 _]
          frame False {
            n263 = property on="CheckList" class="LstBox (strict)"() -> ("Item Symbols"=w425:i32[])  [unwired: 2 in, 2 out]
            n264 = Replace Array Subset(array=w425, new element=w426, index=w427) -> (w424:i32[])
            n265 = property on="CheckList" class="LstBox (strict)"("Item Symbols"=w424) -> ()  [unwired: 2 in, 2 out]
          }
          frame True {
            w428 = 0 ("Top Row")
            n266 = property on="CheckList" class="LstBox (strict)"() -> ("Number of Rows"=w430:u32)  [unwired: 2 in, 2 out]
            n267 = Initialize Array(0, w430) -> (w429:i32[])
            n268 = property on="CheckList" class="LstBox (strict)"("Top Row"=w428, "Value"=w428, "Item Symbols"=w429) -> ()  [unwired: 2 in, 2 out]
          }
        }
      }
      event "CheckList": Key Down {
        # "Update symbols on the listbox\nLeft and right keys check and uncheck"
        n269 = event-data() -> ("VKey"=w435:T20)  [unwired: 1 in]
        n270 = case shown="\"Left\", \"Right\"" w435 {
          selector: w435 -> [w440 _]
          tunnel: eventvkey."Left" ("VKey") -> [w438 _]
          frame "Left", "Right" {
            n271 = Equal?(x=w438, y=w440) -> (x = y?=w439:bool)
            n272 = Select(t=0, s=w439, f=1) -> (s? t:f=w441:i32)
            n273 = property on="CheckList" class="LstBox (strict)"() -> ("Item Symbols"=w444:i32[])  [unwired: 2 in, 2 out]
            n274 = Replace Array Subset(array=w444, new element=w441, index="CheckList") -> (w443:i32[])
            n275 = property on="CheckList" class="LstBox (strict)"("Item Symbols"=w443) -> ()  [unwired: 2 in, 2 out]
          }
          frame Default {
          }
        }
      }
      event "DB Camera Config": Value Change {
        # "Show or hide the cluster of controls, store in ini file"
        n276 = event-data() -> ("NewVal"=w449:bool)  [unwired: 1 in]
        n277 = case shown="False" w449 {
          tunnel: w448 -> [w458 _]
          tunnel: [w451 w469] -> w447
          tunnel: w446 -> [w450 w469]
          frame False {
            w465 = "Camera"
            w468 = FALSE ("Visible")
            n278 = local read "Camera Settings"() -> (w457:T2)
            n279 = Index Array(array=w458) -> (element=w461:cluster{string[]})  [unwired: 1 in]
            n280 = Unbundle(w457) -> ("Frame Rate"=w456:i32, "Compression"=w455:i32, "Size"=w459:u16)
            n281 = Unbundle(w461) -> (w460:string[])
            n282 = Index Array(array=w460, index=w459) -> (element=w454:string)
            n283 = call-poly <vilib>:"Write Key.vi"("section"=w465, "value"=w454, "key"="Size", "refnum"=w450) -> ("refnum out"=w467:T18)  [unwired: 2 in, 5 out]
            n284 = call-poly <vilib>:"Write Key.vi"("section"=w465, "value"=w456, "key"="FrameRate", "refnum"=w467) -> ("refnum out"=w466:T18)  [unwired: 1 in, 6 out]
            n285 = property on="Camera Settings" class="Clust (strict)"("Visible"=w468) -> ()  [unwired: 2 in, 2 out]
            n286 = local write "DB Camera Config"(w468) -> ()
            n287 = call-poly <vilib>:"Write Key.vi"("section"=w465, "value"=w455, "key"="Compression", "refnum"=w466) -> ("refnum out"=w452:T18)  [unwired: 1 in, 6 out]
            n288 = call <vilib>:"Close Config Data.vi"("refnum"=w452) -> ("file path"=w453:path)  [unwired: 2 in, 8 out]
            n289 = call <vilib>:"Open Config Data.vi"("configuration file path"=w453) -> ("refnum"=w451:T18)  [unwired: 8 in, 2 out]
          }
          frame True {
            n290 = property on="Camera Settings" class="Clust (strict)"("Visible"=TRUE) -> ()  [unwired: 2 in, 2 out]
          }
        }
      }
      event "Camera Settings": Value Change {
        # "Update summary string when any elements of DB camera change"
        n291 = event-data() -> ("NewVal"=w483:T2)  [unwired: 1 in]
        n292 = Index Array(array=w479) -> (element=w478:cluster{string[]})  [unwired: 1 in]
        n293 = Unbundle(w483) -> ("Frame Rate"=w474:i32, "Compression"=w473:i32, "Size"=w476:u16)
        n294 = Unbundle(w478) -> (w477:string[])
        n295 = Index Array(array=w477, index=w476) -> (element=w475:string)
        n296 = Format Into String(format string="%s   %dfps   %d%%", w475, w474, w473) -> (resulting string=w480:string)  [unwired: 2 in, 1 out]
        n297 = Build Array(w480) -> (w481:string[])
        n298 = property on="DB Camera Config" class="Bool (strict)"("Strings [4]"=w481) -> ()  [unwired: 2 in, 2 out]
      }
      event "Motor.Enable": Value Change {
        # "When the test mode otor enable helper is set, update that\ntree row item's value"
        n299 = event-data() -> ("NewVal"=w490:bool)  [unwired: 1 in]
        n300 = Unbundle("Motor") -> ("Value"=w489:dbl)  [unwired: 1 out]
        n301 = Select(t=w489, s=w490, f=0.0) -> (s? t:f=w487:dbl)
        n302 = call <vilib>:"NT Write Number.vi"("Numeric"=w487, "Name"=w486) -> ()  [unwired: 9 in, 1 out]
      }
      event "Test Slider": Value Change {
        # "When the test mode slider helper is set, update that\ntree row item's value"
        n303 = event-data() -> ("NewVal"=w494:dbl)  [unwired: 1 in]
        n304 = call <vilib>:"NT Write Number.vi"("Numeric"=w494, "Name"=w495) -> ()  [unwired: 9 in, 1 out]
      }
      event "On/Off": Value Change {
        # "When the test mode on/off helper value is set, update that\ntree row item's value"
        n305 = event-data() -> ("NewVal"=w500:bool)  [unwired: 1 in]
        n306 = Boolean To (0,1)(Boolean=w500) -> (0, 1=w499:i16)
        n307 = call <vilib>:"NT Write Number.vi"("Numeric"=w499, "Name"=w498) -> ()  [unwired: 9 in, 1 out]
      }
      event "Rev/Fwd": Value Change {
        # "When the test mode helper value for relays is set, update that\ntree row item's value"
        n308 = event-data() -> ("NewVal.Forward"=w509:bool, "NewVal.Reverse"=w508:bool)  [unwired: 1 in]
        n309 = Boolean To (0,1)(Boolean=w509) -> (0, 1=w505:i16)
        n310 = Boolean To (0,1)(Boolean=w508) -> (0, 1=w507:i16)
        n311 = Negate(x=w507) -> (-x=w506:i16)
        n312 = Add(x=w505, y=w506) -> (x+y=w504:i16)
        n313 = call <vilib>:"NT Write Number.vi"("Numeric"=w504, "Name"=w503) -> ()  [unwired: 9 in, 1 out]
      }
      event "Test Ring": Value Change {
        # "When a test mode helper value is selected from the ring,\nset the tree item's variable to the string value"
        n314 = event-data() -> ("NewVal"=w514:u16)  [unwired: 1 in]
        n315 = property on="Test Ring" class="Ring (strict)"() -> ("Strings []"=w515:string[])  [unwired: 2 in, 2 out]
        n316 = Index Array(array=w515, index=w514) -> (element=w513:string)
        n317 = call <vilib>:"NT Write String.vi"("String"=w513, "Name"=w512) -> ()  [unwired: 9 in, 1 out]
      }
      event "Rec Mode": Value Change {
        # "Update globals for recording mode and path to read log from.\nClear when logging and let NetworkTables set path for vision to\nuse."
        n318 = event-data() -> ("NewVal"=w527:enum32{"Stop", "Record", "Playback"})  [unwired: 1 in]
        n319 = global write "WPI_DashboardLogging Global.vi" "Logging Filename"(path "") -> ()
        n320 = global write "WPI_DashboardLogging Global.vi" "Recording"(w527) -> ()
        n321 = case shown="\"Playback\"" w527 {
          tunnel: w526 -> [_ w529 w538]
          tunnel: [_ _ w537] -> w523
          tunnel: [_ _ w536] -> _
          tunnel: w521 -> [_ _ w534]
          tunnel: cluster{i32, i32} {-250, 170} -> [_ _ w533]
          tunnel: [_ _ T21 {"Image Size"=TRUE, "Image Type"=TRUE, "Pixel Value"=TRUE, "ROI Information"=TRUE, "Zoom Factor"=FALSE} ("Image Information Shown:All Elements")] -> w519
          tunnel: [_ _ TRUE ("Zoom Factor")] -> w518
          tunnel: w517 -> [_ _ w530]
          frame Default {
          }
          frame "Stop", "Record" {
            # "Place Window too"
            n322 = invoke class="VI" method="FP.Close"(reference=w529) -> (reference out=w528:refnum<vi>)  [unwired: 2 in, 2 out]
            n323 = invoke class="VI" method="Abort VI"(reference=w528) -> ()  [unwired: 2 in, 3 out]
          }
          frame "Playback" {
            n324 = call "Open Playback Panel.vi"("Offset"=w533, "DB VI Ref"=w534, "Playback in"=w538) -> ("Playback out"=w535:refnum<vi>)  [unwired: 8 in]
            n325 = register-events(w535, w530) -> (reference out=w537:refnum<event-registration>, error out=w536:errorcluster)  [unwired: 2 in]
          }
        }
        n326 = property on="Camera Image" class="ImageControl"("Image Information Shown"=w519, "Image Information Visible"=w518) -> ()  [unwired: 2 in, 2 out]
        n327 = call <vilib>:"WPI_DashboardNT Log FieldName Cache.vi"("Operation"=enum16{"Lookup/Add", "Index", "Clear"}."Clear") -> ()  [unwired: 8 in, 3 out]
      }
      event Panel Close {
        w540 = enum32{"Stop", "Record", "Playback"}."Stop" ("Rec Mode")
        # "Playback window has been closed, abort"
        n328 = event-data() -> ()  [unwired: 1 in, 4 out]
        n329 = local write "Rec Mode"(w540) -> ()
        n330 = global write "WPI_DashboardLogging Global.vi" "Recording"(w540) -> ()
      }
      event Panel Close {
        # "Abort playback window and ourself"
        n331 = event-data() -> ()  [unwired: 1 in, 4 out]
        n332 = invoke class="VI" method="FP.Close"(reference=w546) -> (reference out=w545:refnum<vi>)  [unwired: 2 in, 2 out]
        n333 = invoke class="VI" method="Abort VI"(reference=w545) -> (error out=w544:errorcluster)  [unwired: 2 in, 2 out]
        n334 = invoke class="VI" method="Abort VI"(error in=w544) -> ()  [unwired: 2 in, 3 out]
      }
      event User Event {
        n335 = event-data() -> ("IDs"=w554:cluster{"RPC field ID":u16, "Unique ID":u16}, "String"=w553:string)  [unwired: 1 in]
        n336 = Bundle("IDs"=w554, "String"=w553) -> (w552:T9)  [unwired: 1 in]
        n337 = call <vilib>:"Retrieve RPC Response.vi"("RPC Response"=w552) -> ("Output"=w549:string[][])  [unwired: 10 in]
        n338 = Build Array (concatenate)(w547, w549) -> (w548:string[][])
        n339 = local write "Command Params"(w548) -> ()
        n340 = local write "Cmd Status"("" ("Cmd Status")) -> ()
      }
      event "Vision": Value Change {
        # "Enable/Disable Compression slider.\nHW USB is hard-coded into the camera"
        n341 = event-data() -> ("NewVal"=w561:u16)  [unwired: 1 in]
        n342 = Equal?(x=w561, y=u32 2 ("milliseconds to wait")) -> (x = y?=w559:bool)
        n343 = Select(t=T22."Disabled and Grayed Out" ("Disabled"), s=w559, f=T22."Enabled" ("Disabled")) -> (s? t:f=w556:T22)
        n344 = property on="Compression" class="Slide (strict)"("DisabledEnum"=w556) -> ()  [unwired: 2 in, 2 out]
      }
      event "Tree": Double Click {
        n345 = event-data() -> ("PlatMods"=w566:T25, "Tag"=w565:string)  [unwired: 1 in]
        n346 = Unbundle(w566) -> ("Shift"=w564:bool)  [unwired: 4 out]
        n347 = Not(x=w564) -> (.not. x?=w563:bool)
        n348 = call <vilib>:"NT Update Persistence.vi"("Persistence"=w563, "Name"=w565) -> ()  [unwired: 9 in, 1 out]
      }
    }
  }
  n349 = while {
    tunnel: w47 -> [w570]
    i -> [w573]
    stop <- FALSE stop-if-true
    n350 = Wait (ms)(milliseconds to wait=u32 100) -> ()  [unwired: 1 out]
    n351 = case shown="\"Playback\"" "Rec Mode" {
      tunnel: w573 -> [_ _ w588]
      tunnel: [u32 2829099 ("Base Color") u32 11141120 ("Target Color") w577] -> w569
      frame "Stop", Default {
        # "Reset the color, extra updates don't cost much"
      }
      frame "Record" {
      }
      frame "Playback" {
        # "Playback"
        n352 = Quotient & Remainder(x=w588, y=u32 50 ("milliseconds to wait")) -> (x-y*floor(x/y)=w584:u32)  [unwired: 1 out]
        n353 = Divide(x=w584, y=u32 50 ("milliseconds to wait")) -> (x/y=w581:dbl)
        n354 = Multiply(x=6.283185307179586, y=w581) -> (x*y=w586:dbl)
        n355 = Sine(x=w586) -> (sin(x)=w585:dbl)
        n356 = Absolute Value(x=w585) -> (abs(x)=w578:dbl)
        n357 = call "Interpolate RGB Color.vi"("Proportion"=w578, "Target Color"=u32 30976, "Base Color"=u32 2829099) -> ("Result Color"=w577:u32)  [unwired: 8 in]
      }
    }
    n358 = property class="Pane"(reference=w570, "PaneColor"=w569) -> ()  [unwired: 1 in, 2 out]
  }
  n359 = local write "Dashboard Tab"(T1."Teleop" ("Dashboard Tab")) -> ()
  n360 = property on="On/Off" class="Bool (strict)"("Visible"=w15) -> ()  [unwired: 2 in, 2 out]
  n361 = property on="Motor" class="Clust (strict)"("Visible"=w15) -> ()  [unwired: 2 in, 2 out]
  n362 = property on="Progress" class="Clust (strict)"("Visible"=w15) -> ()  [unwired: 2 in, 2 out]
  n363 = property on="Test Ring" class="Ring (strict)"("Visible"=w15) -> ()  [unwired: 2 in, 2 out]
  n364 = property on="Rev/Fwd" class="Clust (strict)"("Visible"=w15) -> ()  [unwired: 2 in, 2 out]
  n365 = property on="Camera Settings" class="Clust (strict)"("Visible"=w15) -> ()  [unwired: 2 in, 2 out]
  n366 = while {
    tunnel: u16 1741 ("timeout ms (25000)") -> [w590]
    stop <- FALSE stop-if-true
    n367 = TCP Create Listener(10:w590) -> (0:w589:errorcluster, 3:w591:refnum<k5>)  [unwired: 4 in, 1 out]
    n368 = case shown="No Error" w589 {
      selector: w589 -> [w593 _]
      tunnel: w591 -> [w594 _]
      frame No Error {
        n369 = while {
          tunnel: w594 -> [w597]
          tunnel: w593 -> [w596]
          stop <- FALSE stop-if-true
          n370 = TCP Wait On Listener(8:w596, 11:w597) -> (0:w598:errorcluster, 4:w599:refnum<k5>)  [unwired: 2 in, 3 out]
          n371 = local write "TCP"(w599) -> ()
          n372 = case shown="No Error" w598 {
            frame No Error {
            }
            frame Error {
              n373 = Wait (ms)(milliseconds to wait=u32 1000) -> ()  [unwired: 1 out]
            }
          }
        }
      }
      frame Error {
        n374 = Wait (ms)(milliseconds to wait=u32 1000) -> ()  [unwired: 1 out]
      }
    }
  }
  n375 = local write "DB Camera Config"(w15) -> ()
  n376 = local write "Command Params"(string[][] [] ("Command Params")) -> ()
  n377 = global write "WPI_DashboardLogging Global.vi" "Recording"(w41) -> ()
  n378 = local write "Command Selection"(u16 0 ("milliseconds to wait")) -> ()
  n379 = local write "Rec Mode"(w41) -> ()
  n380 = disable-structure shown="Disabled" {
    frame Disabled {
      # "There's only one decoration."
      n381 = control-ref of="This VI"() -> (w606:refnum<vi>)
      n382 = property class="VI"(reference=w606) -> (error out=w604:errorcluster, "Panel"=w605:refnum<vi>)  [unwired: 1 in, 1 out]
      n383 = property class="Pnl"(reference=w605, error in=w604) -> ("Decos[]"=w602:refnum<vi>[])  [unwired: 2 out]
      n384 = Index Array(array=w602, index=0) -> (element=w603:refnum<vi>)
      n385 = property class="Decor" props=["Top"](reference=w603) -> ()  [unwired: 2 in, 2 out]
    }
    frame Enabled {
    }
  }
